vi "Read XML to 2D.vi"(8 "error in (no error)":errorcluster, 11 "XML File Path":path) -> (0 "error out":errorcluster, 2 "XML":T1)   [LabVIEW 2011]
doc: "Reads a 2D XML Data style file into a 2D Array\n\nAssumes 6 columns plus variable name\n\n\nVersion 1.0 - 2/14/2010\n\nPhaeron, Inc.\nwww.phaeron.net\n\nMatt Whitlock\n303-669-0310"
uses:
  <vilib>/xml/NI_XML.lvlib
  <libdir>/resource/objmgr/DOMUserDefRef.rc
  <vilib>/xml/Close Reference(Node).vi
  <vilib>/xml/Close Reference(NdList).vi
  <vilib>/xml/Load XML File.vi
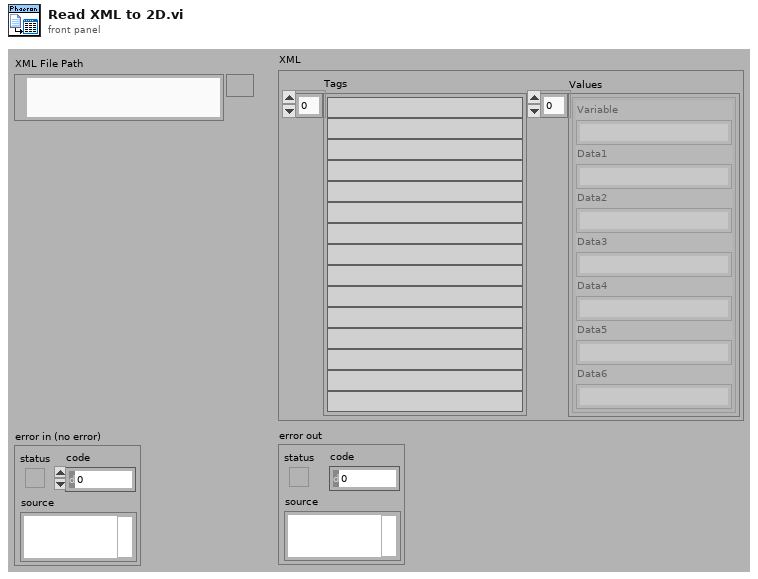
[diagram p1: front panel]
types:
  T1 = cluster{"Tags":string[], "Values":cluster{"Variable":string, "Data1":string, "Data2":string, "Data3":string, "Data4":string, "Data5":string, "Data6":string}[]}
  T2 = cluster{"Variable":string, "Data1":string, "Data2":string, "Data3":string, "Data4":string, "Data5":string, "Data6":string}
  T3 = cluster{string[], cluster{"Variable":string, "Data1":string, "Data2":string, "Data3":string, "Data4":string, "Data5":string, "Data6":string}[]}
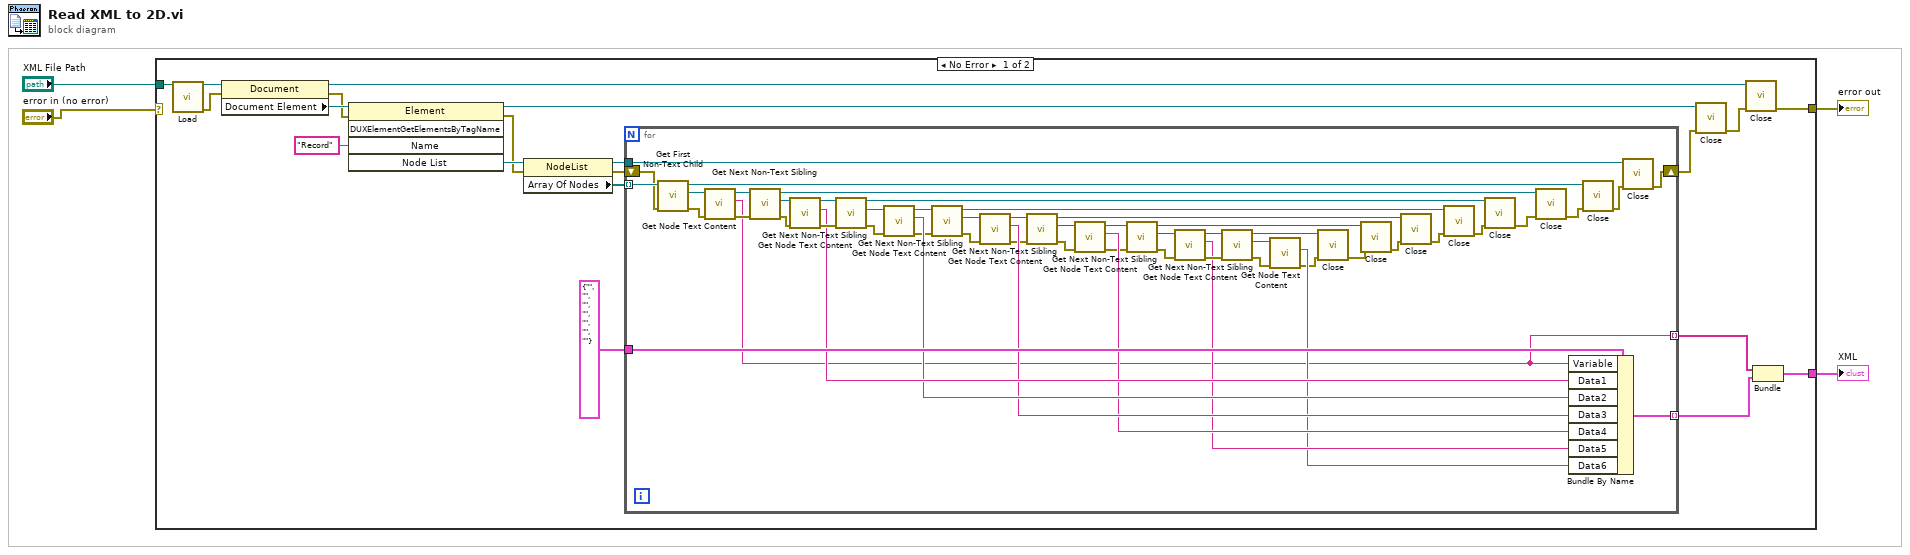
[diagram p0: block diagram]
diagram:
  n1 = case shown="No Error" "error in (no error)" {
    selector: "error in (no error)" -> [_ w79]
    tunnel: "XML File Path" -> [w24 _]
    tunnel: [w9 w79] -> w3
    tunnel: [w8 _] -> w2
    frame No Error {
      n2 = call-poly <vilib>:"Load.vi"("path to XML document"=w24) -> ("DOM document out"=w20:refnum<k20>, "error out"=w23:errorcluster)  [unwired: 12 in, 1 out]
      n3 = property class="Document"(reference=w20, error in=w23) -> (reference out=w12:refnum<k20>, error out=w14:errorcluster, "Document Element"=w22:refnum<k20>)
      n4 = invoke class="Element" method="DUXElementGetElementsByTagName"(reference=w22, error in=w14, "Name"="Record" ("Tag Name")) -> (reference out=w11:refnum<k20>, error out=w15:errorcluster, "Node List"=w19:refnum<k20>)  [unwired: 2 in, 2 out]
      n5 = property class="NodeList"(reference=w19, error in=w15) -> (reference out=w17:refnum<k20>, error out=w16:errorcluster, "Array Of Nodes"=w18:refnum<k20>[])
      n6 = for {
        tunnel: w18 -> [w75] mode=indexing
        tunnel: w17 -> [w78]
        shift-right: [w71] -> w10
        shift-left: w16 -> [w74]
        tunnel: T2 {"Variable"="", "Data1"="", "Data2"="", "Data3"="", "Data4"="", "Data5"="", "Data6"=""} ("Data Dictionary") -> [w70]
        tunnel: [w69] -> w7 mode=indexing
        tunnel: [w25] -> w6 mode=indexing
        n7 = call <vilib>:"Get First Non-Text Child.vi"("error in (no error)"=w74, "node in"=w75) -> ("error out"=w77:errorcluster, "child node"=w76:refnum<k20>, "node out"=w73:refnum<k20>)  [unwired: 7 out]
        n8 = call <vilib>:"Get Node Text Content.vi"("error in (no error)"=w77, "node in"=w76) -> ("error out"=w58:errorcluster, "node text"=w25:string, "node out"=w59:refnum<k20>)  [unwired: 7 out]
        n9 = call <vilib>:"Get Next Non-Text Sibling.vi"("error in (no error)"=w58, "node in"=w59) -> ("error out"=w60:errorcluster, "sibling node"=w61:refnum<k20>, "node out"=w62:refnum<k20>)  [unwired: 7 out]
        n10 = call <vilib>:"Get Node Text Content.vi"("error in (no error)"=w60, "node in"=w61) -> ("error out"=w66:errorcluster, "node text"=w57:string, "node out"=w64:refnum<k20>)  [unwired: 7 out]
        n11 = call <vilib>:"Get Next Non-Text Sibling.vi"("error in (no error)"=w66, "node in"=w64) -> ("error out"=w67:errorcluster, "sibling node"=w68:refnum<k20>, "node out"=w65:refnum<k20>)  [unwired: 7 out]
        n12 = call <vilib>:"Get Node Text Content.vi"("error in (no error)"=w67, "node in"=w68) -> ("error out"=w50:errorcluster, "node text"=w56:string, "node out"=w53:refnum<k20>)  [unwired: 7 out]
        n13 = call <vilib>:"Get Next Non-Text Sibling.vi"("error in (no error)"=w50, "node in"=w53) -> ("error out"=w55:errorcluster, "sibling node"=w54:refnum<k20>, "node out"=w52:refnum<k20>)  [unwired: 7 out]
        n14 = call <vilib>:"Get Node Text Content.vi"("error in (no error)"=w55, "node in"=w54) -> ("error out"=w45:errorcluster, "node text"=w49:string, "node out"=w46:refnum<k20>)  [unwired: 7 out]
        n15 = call <vilib>:"Get Next Non-Text Sibling.vi"("error in (no error)"=w45, "node in"=w46) -> ("error out"=w47:errorcluster, "sibling node"=w48:refnum<k20>, "node out"=w43:refnum<k20>)  [unwired: 7 out]
        n16 = call <vilib>:"Get Node Text Content.vi"("error in (no error)"=w47, "node in"=w48) -> ("error out"=w33:errorcluster, "node text"=w44:string, "node out"=w34:refnum<k20>)  [unwired: 7 out]
        n17 = call <vilib>:"Get Next Non-Text Sibling.vi"("error in (no error)"=w33, "node in"=w34) -> ("error out"=w35:errorcluster, "sibling node"=w36:refnum<k20>, "node out"=w37:refnum<k20>)  [unwired: 7 out]
        n18 = call <vilib>:"Get Node Text Content.vi"("error in (no error)"=w35, "node in"=w36) -> ("error out"=w41:errorcluster, "node text"=w32:string, "node out"=w40:refnum<k20>)  [unwired: 7 out]
        n19 = call <vilib>:"Get Next Non-Text Sibling.vi"("error in (no error)"=w41, "node in"=w40) -> ("error out"=w39:errorcluster, "sibling node"=w38:refnum<k20>, "node out"=w42:refnum<k20>)  [unwired: 7 out]
        n20 = call <vilib>:"Get Node Text Content.vi"("error in (no error)"=w39, "node in"=w38) -> ("error out"=w30:errorcluster, "node text"=w31:string)  [unwired: 8 out]
        n21 = call-poly <vilib>:"Close.vi"("error in (no error)"=w30, "node"=w42) -> ("error out"=w29:errorcluster)  [unwired: 7 out]
        n22 = call-poly <vilib>:"Close.vi"("error in (no error)"=w29, "node"=w37) -> ("error out"=w28:errorcluster)  [unwired: 7 out]
        n23 = call-poly <vilib>:"Close.vi"("error in (no error)"=w28, "node"=w43) -> ("error out"=w27:errorcluster)  [unwired: 7 out]
        n24 = call-poly <vilib>:"Close.vi"("error in (no error)"=w27, "node"=w52) -> ("error out"=w26:errorcluster)  [unwired: 7 out]
        n25 = call-poly <vilib>:"Close.vi"("error in (no error)"=w26, "node"=w65) -> ("error out"=w63:errorcluster)  [unwired: 7 out]
        n26 = call-poly <vilib>:"Close.vi"("error in (no error)"=w63, "node"=w62) -> ("error out"=w51:errorcluster)  [unwired: 7 out]
        n27 = Bundle By Name(cluster=w70, "Variable"=w25, "Data1"=w57, "Data2"=w56, "Data3"=w49, "Data4"=w44, "Data5"=w32, "Data6"=w31) -> (w69:T2)
        n28 = call-poly <vilib>:"Close.vi"("error in (no error)"=w51, "node"=w73) -> ("error out"=w72:errorcluster)  [unwired: 7 out]
        n29 = call-poly <vilib>:"Close.vi"("error in (no error)"=w72, "node list"=w78) -> ("error out"=w71:errorcluster)  [unwired: 7 out]
      }
      n30 = call-poly <vilib>:"Close.vi"("error in (no error)"=w10, "node"=w11) -> ("error out"=w13:errorcluster)  [unwired: 7 out]
      n31 = call-poly <vilib>:"Close.vi"("error in (no error)"=w13, "node"=w12) -> ("error out"=w9:errorcluster)  [unwired: 7 out]
      n32 = Bundle(w6, w7) -> (w8:T3)  [unwired: 1 in]
    }
    frame Error {
    }
  }
  "error out" <- w3
  "XML" <- w2
